vi "Initialization VI.vi"(8 "error in (no error)":errorcluster, 10 "Custom XML":string, 11 "Device Item Ref in":T1 format="%.0x") -> (0 "error out":errorcluster, 3 "Device Item Ref out":T1 format="%.0x")   [LabVIEW 2019, in "DeltaPSControl System Explorer.lvlib"]
uses:
  DeltaPSControl System Explorer.lvlib
  <vilib>/NI VeriStand/Custom Device API/Custom Device Item Ref.ctl
  <vilib>/NI VeriStand/Custom Device API/Custom Device Channel.ctl
  <vilib>/NI VeriStand/Custom Device API/Custom Device Channel Type.ctl
  Shared/Constants.vi
  <vilib>/NI VeriStand/Custom Device API/Custom Device API.lvlib
  Shared/DeltaPSControl Shared.lvlib
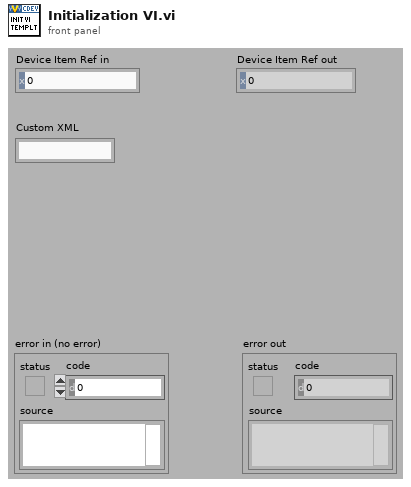
[diagram p1: front panel]
types:
  T1 = typedef "Custom Device API.lvlib/Custom Device Item Ref.ctl" = u64
  T2 = typedef "Custom Device API.lvlib/Custom Device Channel.ctl" = cluster{"Type":T3, "Units":string, "Default Value":dbl, "Faultable":bool, "Scalable":bool}
  T3 = typedef "Custom Device API.lvlib/Custom Device Channel Type.ctl" = enum16{"Input", "Output"}
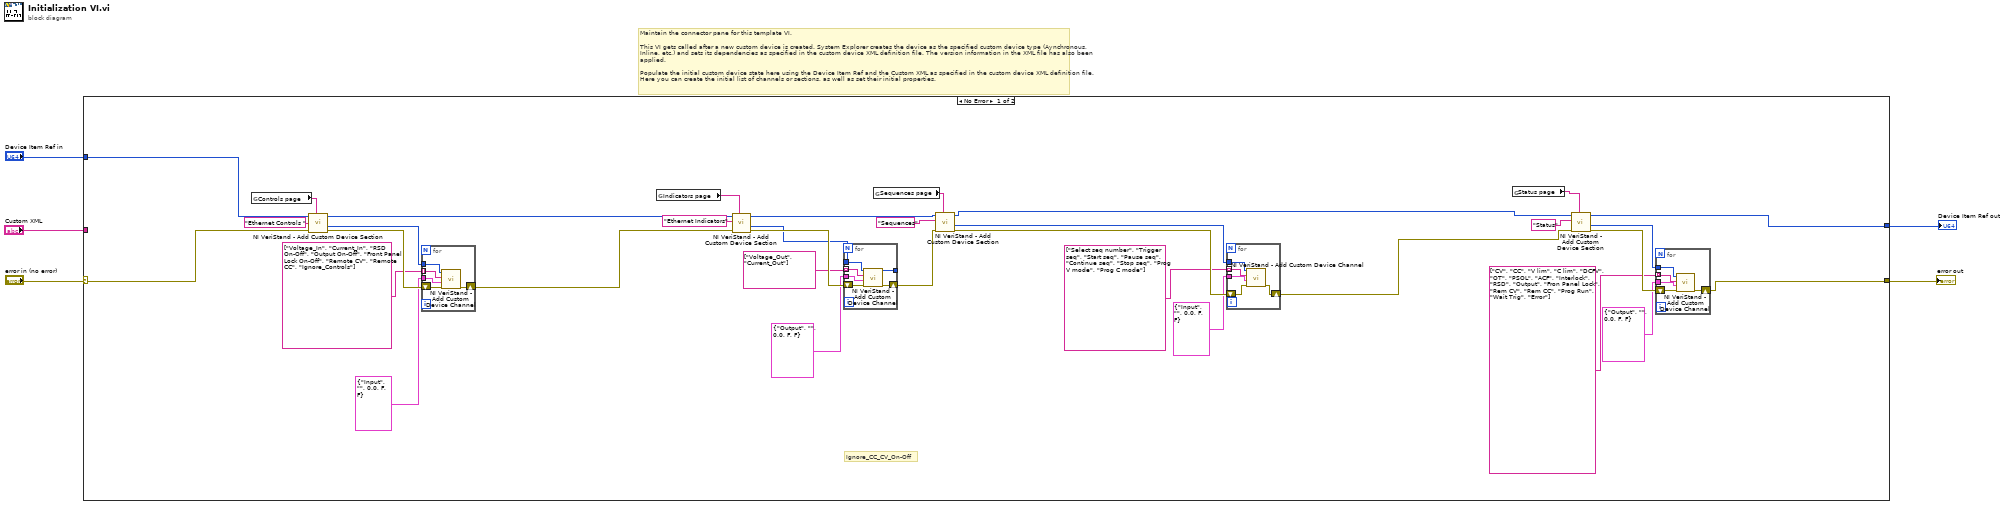
[diagram p0: block diagram]
diagram:
  # "Maintain the connector pane for this template VI.\n\nThis VI gets called after a new custom device is created. System Explorer creates the device as the specified custom device type (Aynchronous, Inline, etc.) and sets its dependencies as specified in the custom device XML definition file. The version information in the XML file has also been applied.\n\nPopulate the initial custom device state here using the Device Item Ref and the Custom XML as specified in the custom device XML definition file. Here you can create the initial list of channels or sections, as well as set their initial properties."
  n1 = case shown="No Error" "error in (no error)" {
    selector: "error in (no error)" -> [w13 w62]
    tunnel: [w6 w62] -> w5
    tunnel: [w7 w61] -> w3
    tunnel: "Device Item Ref in" -> [w12 w61]
    tunnel: "Custom XML" -> [_ _]
    frame No Error {
      # "Ignore_CC_CV_On-Off"
      n2 = global read "Constants.vi" "Controls page"() -> (w11:string)
      n3 = call <vilib>:"NI VeriStand - Add Custom Device Section.vi"("GUID (Default Section)"=w11, "error in (no error)"=w13, "Section Name"="Ethernet Controls ", "Parent Ref in"=w12) -> ("error out"=w29:errorcluster, "Section Ptr"=w30:T1, "Parent Ref out"=w26:T1)  [unwired: 4 in, 1 out]
      n4 = for {
        tunnel: w30 -> [w55]
        shift-right: [w53] -> w39
        shift-left: w29 -> [w54]
        tunnel: T2 {"Type"=enum."Input", "Units"="", "Default Value"=0.0, "Faultable"=FALSE, "Scalable"=FALSE} ("Channel") -> [w52]
        tunnel: string[] ["Voltage_In", "Current_In", "RSD On-Off", "Output On-Off", "Front Panel Lock On-Off", "Remote CV", "Remote CC", "Ignore_Controls"] -> [w51] mode=indexing
        n5 = call <vilib>:"NI VeriStand - Add Custom Device Channel.vi"("error in (no error)"=w54, "Channel"=w52, "Channel Name"=w51, "Parent Ref in"=w55) -> ("error out"=w53:errorcluster)  [unwired: 4 in, 3 out]
      }
      n6 = global read "Constants.vi" "Indicators page"() -> (w10:string)
      n7 = call <vilib>:"NI VeriStand - Add Custom Device Section.vi"("GUID (Default Section)"=w10, "error in (no error)"=w39, "Section Name"="Ethernet Indicators", "Parent Ref in"=w26) -> ("error out"=w33:errorcluster, "Section Ptr"=w31:T1, "Parent Ref out"=w32:T1)  [unwired: 4 in, 1 out]
      n8 = for {
        tunnel: w31 -> [w50]
        shift-right: [w48] -> w34
        shift-left: w33 -> [w49]
        tunnel: T2 {"Type"=enum."Output", "Units"="", "Default Value"=0.0, "Faultable"=FALSE, "Scalable"=FALSE} ("Channel") -> [w47]
        tunnel: string[] ["Voltage_Out", "Current_Out"] -> [w46] mode=indexing
        tunnel: [w45] -> _
        n9 = call <vilib>:"NI VeriStand - Add Custom Device Channel.vi"("error in (no error)"=w49, "Channel"=w47, "Channel Name"=w46, "Parent Ref in"=w50) -> ("error out"=w48:errorcluster, "Parent Ref out"=w45:T1)  [unwired: 4 in, 2 out]
      }
      n10 = global read "Constants.vi" "Sequences page"() -> (w9:string)
      n11 = call <vilib>:"NI VeriStand - Add Custom Device Section.vi"("GUID (Default Section)"=w9, "error in (no error)"=w34, "Section Name"="Sequences", "Parent Ref in"=w32) -> ("error out"=w36:errorcluster, "Section Ptr"=w35:T1, "Parent Ref out"=w37:T1)  [unwired: 4 in, 1 out]
      n12 = for {
        tunnel: w35 -> [w44]
        shift-right: [w42] -> w38
        shift-left: w36 -> [w43]
        tunnel: T2 {"Type"=enum."Input", "Units"="", "Default Value"=0.0, "Faultable"=FALSE, "Scalable"=FALSE} ("Channel") -> [w41]
        tunnel: string[] ["Select seq number", "Trigger seq", "Start seq", "Pause seq", "Continue seq", "Stop seq", "Prog V mode", "Prog C mode"] ("appended array") -> [w40] mode=indexing
        n13 = call <vilib>:"NI VeriStand - Add Custom Device Channel.vi"("error in (no error)"=w43, "Channel"=w41, "Channel Name"=w40, "Parent Ref in"=w44) -> ("error out"=w42:errorcluster)  [unwired: 4 in, 3 out]
      }
      n14 = global read "Constants.vi" "Status page"() -> (w8:string)
      n15 = call <vilib>:"NI VeriStand - Add Custom Device Section.vi"("GUID (Default Section)"=w8, "error in (no error)"=w38, "Section Name"="Status", "Parent Ref in"=w37) -> ("error out"=w28:errorcluster, "Section Ptr"=w27:T1, "Parent Ref out"=w7:T1)  [unwired: 4 in, 1 out]
      n16 = for {
        tunnel: w27 -> [w60]
        shift-right: [w58] -> w6
        shift-left: w28 -> [w59]
        tunnel: T2 {"Type"=enum."Output", "Units"="", "Default Value"=0.0, "Faultable"=FALSE, "Scalable"=FALSE} ("Channel") -> [w57]
        tunnel: string[] ["CV", "CC", "V lim", "C lim", "DCFV", "OT", "PSOL", "ACF", "Interlock", "RSD", "Output", "Fron Panel Lock", "Rem CV", "Rem CC", "Prog Run", "Wait Trig", "Error"] -> [w56] mode=indexing
        n17 = call <vilib>:"NI VeriStand - Add Custom Device Channel.vi"("error in (no error)"=w59, "Channel"=w57, "Channel Name"=w56, "Parent Ref in"=w60) -> ("error out"=w58:errorcluster)  [unwired: 4 in, 3 out]
      }
    }
    frame Error {
    }
  }
  "error out" <- w5
  "Device Item Ref out" <- w3
